vi "AI-204 Acquire  Chart PointByPoint Current with Circuit Breaker Control.vi"() -> ()   [LabVIEW 8.6]
uses:
  <vilib>/UeiDaq/UeiDaqConfigureTimingForSimpleIO.vi
  <libdir>/resource/objmgr/UeiDaq.rc
  <vilib>/UeiDaq/UeiDaqCreateAICurrentSession.vi
  <vilib>/UeiDaq/UeiDaqReadOneScaledScan.vi
panel:
  in  "CB enable":i32[](array[ring]) items=["Disabled", "Enabled", "Auto"]
  in  "Maximum range":dbl(ring) items=["0.025", "0.0125", "0.005", "0.0025"]
  in  "Minimum range":dbl(ring) items=["-0.025", "-0.0125", "-0.005", "-0.0025"]
  out "Tripped channels":bool[](array[boolean])
  out "CB Status Mask":u32
  in  "Reset CB":bool
  in  "timeout (ms)":u32
  in  "Analog Input Mode":enum16{"Differential", "Single-Ended"}(ring)
  in  "Resource":string
  out "Total scans acquired":u32
  out "Waveform Chart":dbl[][](graph)
  in  "Refresh rate (ms)":u32
  in  "stop":bool
  # "AI-204 Software timed analog input acquisition with circuit breaker control"
  # "This Example takes an input current and graphs it over time.  There are maximum and minimum\nlimits for the input current that allows the user to utilize the CB function of the AI-204."
  # "0"
  # "1"
  # "There  are  three  modes  that  the  CB can be configured  in,  Disabled,  Enabled  and  Auto.  In \nDisabled mode, if the input current exceeds the specified input range, the current measurement \nwill  clip  to the  maximum or  minimum  range  value.   In Enabled  mode,  If  the  input current \nexceeds  the specified  input  range for  longer than  100ms, the  circuit  breaker will disconnect \nthe circuit  to protect  input  resistors  from overcurrent.  In Auto  mode,  the  CB  status  is set in \nPowerDNA Explorer to either Enabled or Disabled and saved in the EEPROM."
  # "2"
  # "3"
  # "4"
  # "5"
  # "6"
  # "7"
  # "8"
  # "9"
  # "10"
  # "11"
  # "12"
  # "13"
  # "14"
  # "15"
  # "16"
  # "17"
  # "18"
  # "19"
  # "20"
  # "21"
  # "22"
  # "23"
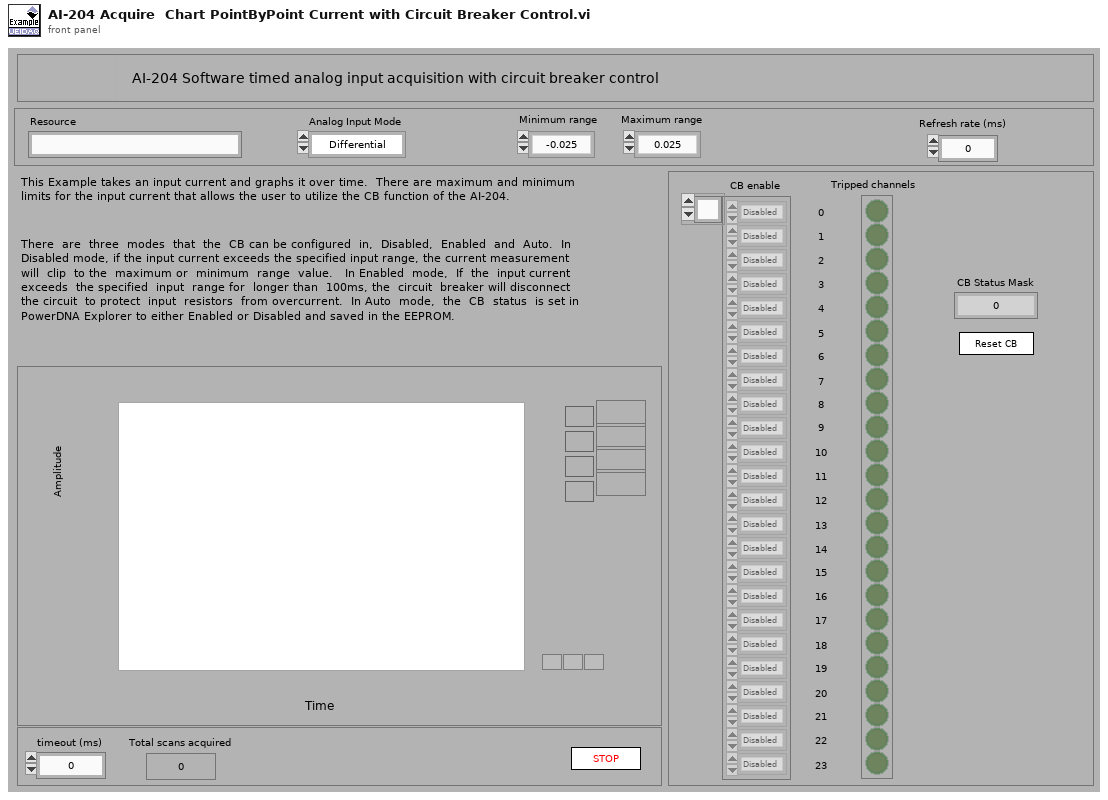
[diagram p1: front panel]
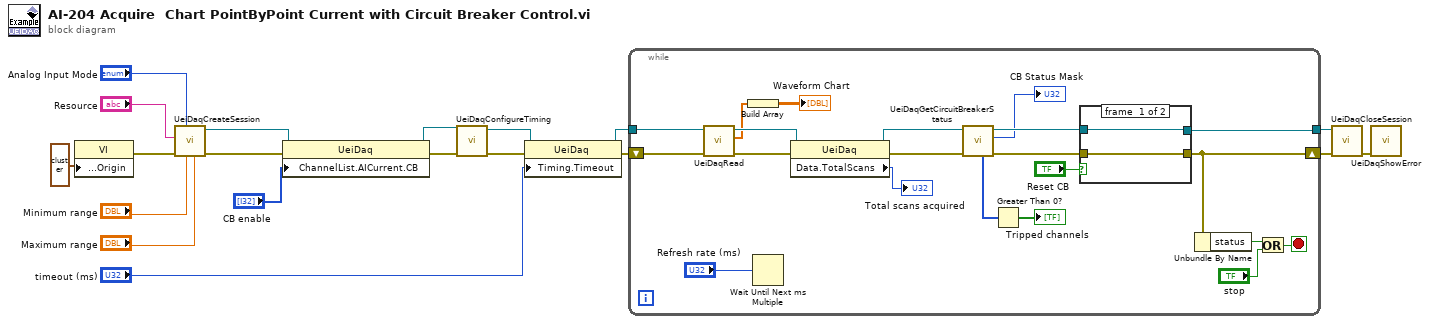
[diagram p0: block diagram]
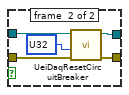
[diagram p2: hidden frame]
diagram:
  n1 = property class="VI"("Front Panel.Origin"=cluster{"Horizontal":i16, "Vertical":i16} ? ("Front Panel Window:Origin")) -> (error out=w14:errorcluster)  [unwired: 2 in, 1 out]
  n2 = call-poly <vilib>:"UeiDaqCreateSession.vi"("Maximum range"="Maximum range", "Minimum range"="Minimum range", "Analog Input Mode"="Analog Input Mode", "error in (no error)"=w14, "Resource"="Resource") -> ("error out"=w7:errorcluster, "UeiDaq Refnum Out"=w5:refnum<k20>)  [unwired: 2 in, 3 out]
  n3 = property class="UeiDaq"(reference=w5, error in=w7, "ChannelList.AICurrent.CB"="CB enable") -> (reference out=w4:refnum<k20>, error out=w6:errorcluster)
  n4 = call-poly <vilib>:"UeiDaqConfigureTiming.vi"("error in (no error)"=w6, "UeiDaq Refnum In"=w4) -> ("error out"=w12:errorcluster, "UeiDaq Refnum Out"=w10:refnum<k20>)  [unwired: 1 in, 7 out]
  n5 = property class="UeiDaq"(reference=w10, error in=w12, "Timing.Timeout"="timeout (ms)") -> (reference out=w9:refnum<k20>, error out=w11:errorcluster)
  n6 = while {
    tunnel: w9 -> [w37]
    tunnel: [w26] -> w18
    shift-right: [w23] -> w17
    shift-left: w11 -> [w24]
    stop <- w38 stop-if-true
    n7 = call-poly <vilib>:"UeiDaqRead.vi"("error in (no error)"=w24, "UeiDaq Refnum In"=w37) -> ("error out"=w34:errorcluster, "Scaled Data"=w32:dbl[], "UeiDaq Refnum Out"=w35:refnum<k20>)  [unwired: 7 out]
    n8 = Build Array(w32) -> (→"Waveform Chart":dbl[][])
    n9 = Wait Until Next ms Multiple(millisecond multiple="Refresh rate (ms)") -> ()  [unwired: 1 out]
    n10 = property class="UeiDaq"(reference=w35, error in=w34) -> (reference out=w30:refnum<k20>, error out=w29:errorcluster, "Data.TotalScans"=→"Total scans acquired":u32)
    n11 = call <vilib>:"UeiDaqGetCircuitBreakerStatus.vi"("error in (no error)"=w29, "UeiDaq Refnum In"=w30) -> ("error out"=w27:errorcluster, "Current Status Mask"=→"CB Status Mask":u32, "UeiDaq Refnum Out"=w28:refnum<k20>, "Detailed Status Per Channel"=w21:u32[])  [unwired: 6 out]
    n12 = Greater Than 0?(x=w21) -> (x > 0?=→"Tripped channels":bool[])
    n13 = case shown="True" "Reset CB" {
      tunnel: w28 -> [w42 w47]
      tunnel: w27 -> [w41 w46]
      tunnel: [w42 w45] -> w26
      tunnel: [w41 w44] -> w23
      frame #0 {
      }
      frame #1 {
        n14 = call <vilib>:"UeiDaqResetCircuitBreaker.vi"("error in (no error)"=w46, "Reset Mask"=u32 ?, "UeiDaq Refnum In"=w47) -> ("error out"=w44:errorcluster, "UeiDaq Refnum Out"=w45:refnum<k20>)  [unwired: 7 out]
      }
    }
    n15 = Unbundle By Name(w23) -> ("status"=w40:bool)
    n16 = Or(x=w40, y="stop") -> (x .or. y?=w38:bool)
  }
  n17 = call <vilib>:"UeiDaqCloseSession.vi"("error in (no error)"=w17, "UeiDaq Refnum In"=w18) -> ("error out"=w19:errorcluster)  [unwired: 1 in, 8 out]
  n18 = call <vilib>:"UeiDaqShowError.vi"("error in (no error)"=w19) -> ()  [unwired: 1 in, 10 out]
